vi "SetGearMainpulatorUpDown.vi"   [LabVIEW 2016, in "Gear Manipulator.lvclass"]
uses:
  Gear Manipulator.lvclass
  Gear Manipulator.lvclass/Gear Manipulator.ctl
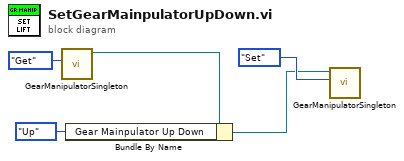
[diagram p0: block diagram]
diagram:
  n1 = call "GearManipulatorSingleton.vi"("Get/Set"=enum16{"Get", "Set"}."Get") -> ("Gear Manipulator.lvclass"=w1:refnum<class "Gear Manipulator.lvclass">)  [unwired: 9 in, 1 out]
  n2 = Bundle By Name(cluster=w1, "Gear Mainpulator Up Down"=enum16{"Up", "Down"}."Up") -> (w2:refnum<class "Gear Manipulator.lvclass">)
  n3 = call "GearManipulatorSingleton.vi"("Get/Set"=enum16{"Get", "Set"}."Set", "Gear Manipulator.lvclass"=w2) -> ()  [unwired: 8 in, 2 out]
